vi "PI_Scanner_In_Range.vi"(0 "Picture size":dbl=50.0 min=0.1 max=200.0 format="%1.1f um", 1 "Picture size 2":dbl=50.0 min=0.1 max=200.0 format="%1.1f um", 4 "Upper Left":T1, 7 "Axis":enum32{"x-y", "x-z", "y-z"}(ring)) -> (14 "Picture size out":dbl=50.0 min=0.1 max=200.0 format="%1.1f um", 15 "Picture size out 2":dbl=50.0 min=0.1 max=200.0 format="%1.1f um")   [LabVIEW 2013]
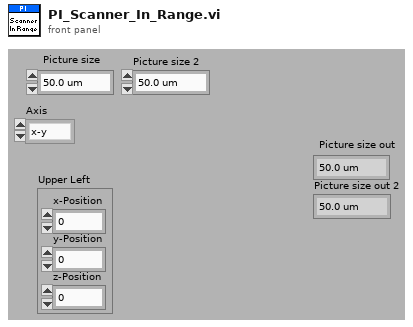
[diagram p1: front panel]
types:
  T1 = cluster{"x-Position":dbl, "y-Position":dbl, "z-Position":dbl}
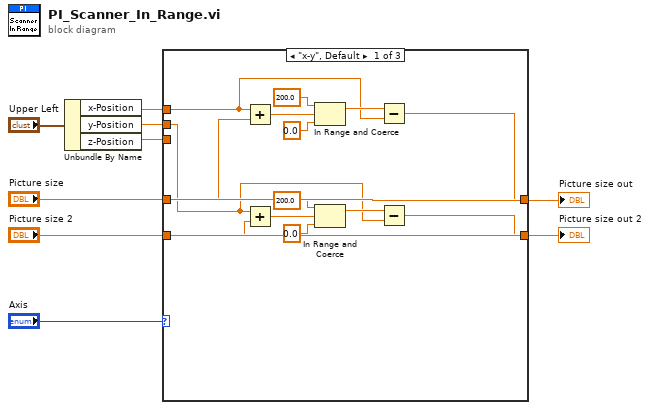
[diagram p0: block diagram]
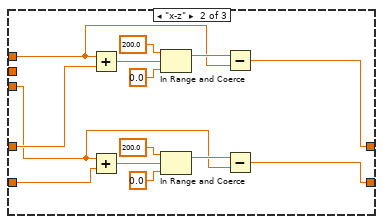
[diagram p2: hidden frame]
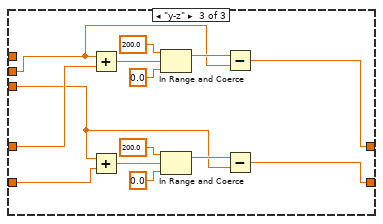
[diagram p3: hidden frame]
diagram:
  n1 = Unbundle By Name("Upper Left") -> ("x-Position"=w2:dbl, "y-Position"=w3:dbl, "z-Position"=w1:dbl)
  n2 = case shown="\"x-y\", Default" "Axis" {
    tunnel: "Picture size" -> [w21 w35 w49]
    tunnel: "Picture size 2" -> [w20 w34 w48]
    tunnel: w3 -> [w10 _ w36]
    tunnel: w2 -> [w11 w25 _]
    tunnel: w1 -> [_ w22 w37]
    tunnel: [w9 w24 w39] -> _
    tunnel: [w8 w23 w38] -> _
    frame "x-y", Default {
      n3 = Add(x=w11, y=w21) -> (x+y=w19:dbl)
      n4 = Add(x=w10, y=w20) -> (x+y=w18:dbl)
      n5 = In Range and Coerce(upper limit=200.0, x=w19, lower limit=0.0) -> (coerced(x)=w13:dbl)  [unwired: 1 out]
      n6 = In Range and Coerce(upper limit=200.0, x=w18, lower limit=0.0) -> (coerced(x)=w12:dbl)  [unwired: 1 out]
      n7 = Subtract(x=w13, y=w11) -> (x-y=w9:dbl)
      n8 = Subtract(x=w12, y=w10) -> (x-y=w8:dbl)
    }
    frame "x-z" {
      n9 = Add(x=w25, y=w35) -> (x+y=w33:dbl)
      n10 = Add(x=w22, y=w34) -> (x+y=w32:dbl)
      n11 = In Range and Coerce(upper limit=200.0, x=w33, lower limit=0.0) -> (coerced(x)=w27:dbl)  [unwired: 1 out]
      n12 = In Range and Coerce(upper limit=200.0, x=w32, lower limit=0.0) -> (coerced(x)=w26:dbl)  [unwired: 1 out]
      n13 = Subtract(x=w27, y=w25) -> (x-y=w24:dbl)
      n14 = Subtract(x=w26, y=w22) -> (x-y=w23:dbl)
    }
    frame "y-z" {
      n15 = Add(x=w36, y=w49) -> (x+y=w47:dbl)
      n16 = Add(x=w37, y=w48) -> (x+y=w46:dbl)
      n17 = In Range and Coerce(upper limit=200.0, x=w47, lower limit=0.0) -> (coerced(x)=w41:dbl)  [unwired: 1 out]
      n18 = In Range and Coerce(upper limit=200.0, x=w46, lower limit=0.0) -> (coerced(x)=w40:dbl)  [unwired: 1 out]
      n19 = Subtract(x=w41, y=w36) -> (x-y=w39:dbl)
      n20 = Subtract(x=w40, y=w37) -> (x-y=w38:dbl)
    }
  }
  "Picture size out" <- "Picture size"
  "Picture size out 2" <- "Picture size 2"
